vi "Test_LogtoNestedGlobalLogInstance_LogCapturedInGlobalLog.vi"(8 "error in (no error)":errorcluster, 11 "TestCase in":refnum<class "TestComposedLog.lvclass">) -> (0 "error out":errorcluster, 3 "TestCase out":refnum<class "TestComposedLog.lvclass">)   [LabVIEW 2017, in "TestComposedLog.lvclass"]
uses:
  TestComposedLog.lvclass
  Source/Composed Log/Types/Log Level.ctl
  Source/LVQueue Sink/LVQueue Sink.lvclass/LVQueue Sink.ctl
  Source/Composed Log/LoggerReference/LoggerReference.lvclass/LoggerReference.ctl
  26ac907e-b197-4f92-b50b-edca335a3ee8.vi
  26ac907e-b197-4f92-b50b-edca335a3ee8.vi/98f69271-1de1-4081-8ac1-8b840b0807ac.vi
  Source/Composed Log/Singleton Event Log/Get Nested Global Log Instance.vi/b2f05d58-65df-4e80-8f90-78513ac31376.vi
  Source/Composed Log/LoggerReference/Log.vi
  Source/Composed Log/LoggerReference/Get Valid Event Time.vi
  Source/Composed Log/LoggerReference/Return Aggregate Queues.vi
  Source/Composed Log/LoggerReference/Add Aggregate Log.vi
  26ac907e-b197-4f92-b50b-edca335a3ee8.vi/98f69271-1de1-4081-8ac1-8b840b0807ac.vi/bbd2f978-e444-4445-9202-4eeb40a61ae4.vi
  Source/Composed Log/Singleton Event Log/Get Nested Global Log Instance.vi/b2f05d58-65df-4e80-8f90-78513ac31376.vi/e1ecde32-be62-4caa-aa7a-1c02d969ae2d.vi
  Source/Composed Log/LoggerReference/Remove Stale Logs.vi
  Source/Composed Log/LoggerReference/Send Add Sink.vi
  Source/LVQueue Sink/LVQueue Sink.lvclass
  C:/CS/Internal/LabVIEW/Logger/Source/Composed Log/Log Sink/Log Sink.lvclass
  Source/Composed Log/Application Logger/Launch Worker Loop.vi
  Source/Composed Log/LoggerReference/Initialize Logger Instance.vi
  Source/Composed Log/Singleton Event Log/Logger Queue FGV.vi
  Source/Composed Log/Singleton Event Log/Shared Instance FGV.vi
  Source/Composed Log/IErrorFormat/IErrorFormat.lvclass
  Source/Composed Log/LoggerReference/LoggerReference.lvclass
  Source/Composed Log/Log Sink/Log Sink.lvclass
  <vilib>/addons/_JKI Toolkits/VI Tester/TestCase.llb/TestCase.lvclass
  Source/Composed Log/Composed Log.lvlib
  Source/Composed Log/Singleton Event Log/Singleton Event Log.lvlib
  C:/Program Files (x86)/National Instruments/LabVIEW 2017/vi.lib/addons/_JKI Toolkits/VI Tester/TestCase.llb/TestCase.lvclass
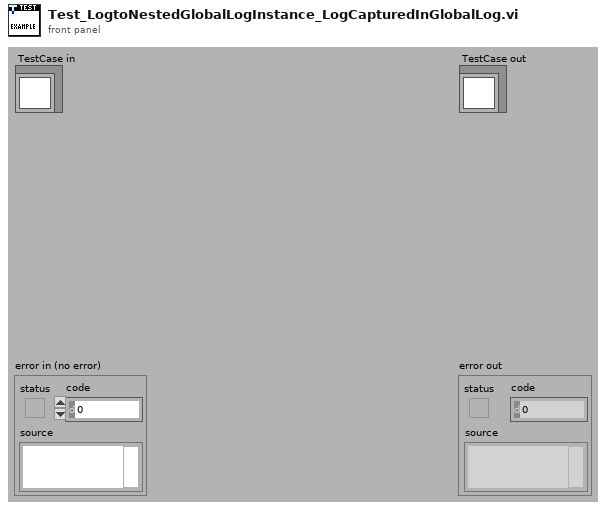
[diagram p1: front panel]
types:
  T1 = typedef "Composed Log.lvlib/Log Level.ctl" = enum16{"Debug", "Info", "Warning", "Error", "Critical"}
  T2 = typedef "Composed Log.lvlib/Log Packet.ctl" = cluster{"Data To Log":string, "Source":string, "Event Level":T1, "Event Time":timestamp}
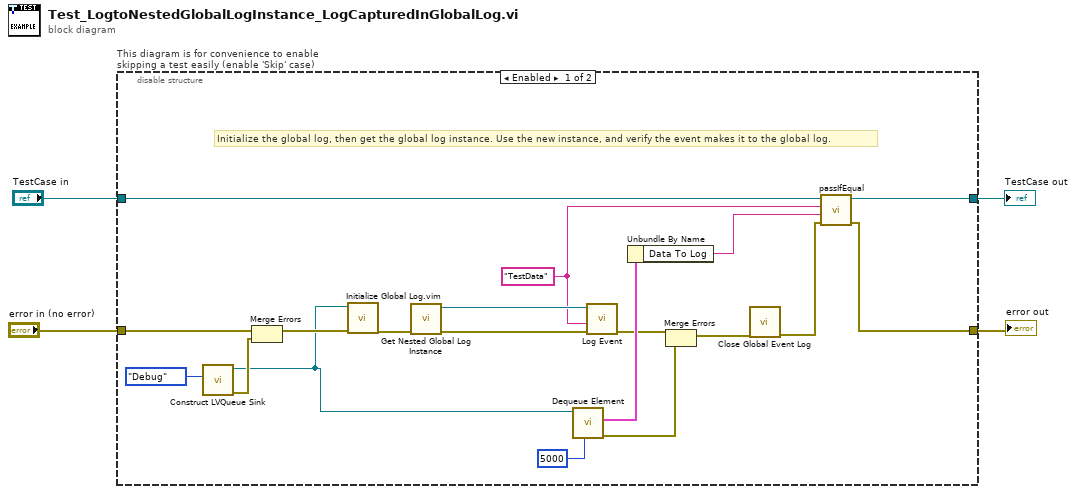
[diagram p0: block diagram]
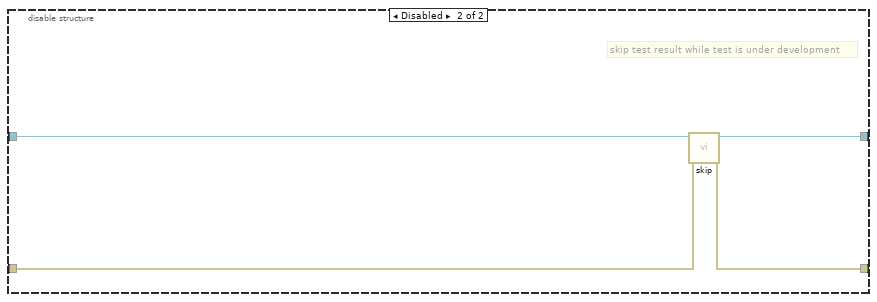
[diagram p2: hidden frame]
diagram:
  n1 = disable-structure "This diagram is for convenience to enable skipping a test easily (enable 'Skip' case)" shown="Enabled" {
    disable-tunnel: "TestCase in" -> [w18 w27]
    disable-tunnel: [w15 w25] -> w1
    disable-tunnel: [w16 w26] -> w3
    disable-tunnel: "error in (no error)" -> [w23 w24]
    frame Enabled {
      w6 = "TestData" ("Data To Log")
      # "Initialize the global log, then get the global log instance. Use the new instance, and verify the event makes it to the global log."
      n2 = call "Construct LVQueue Sink.vi"("LogLevel"=Log_Level."Debug") -> ("error out"=w21:errorcluster, "LVQueue Sink out"=w13:refnum<class "LVQueue Sink.lvclass">)  [unwired: 9 in]
      n3 = Merge Errors(w23, w21) -> (w20:errorcluster)
      n4 = call "Initialize Global Log.vim"("error in (no error)"=w20, "Log Sink(s)"=w13) -> ("error out"=w19:errorcluster)  [unwired: 8 in, 1 out]
      n5 = call "Get Nested Global Log Instance.vi"("error in (no error)"=w19) -> ("error out"=w8:errorcluster, "Nested Global Log Instance Reference"=w7:refnum<class "LoggerReference.lvclass">)  [unwired: 9 in]
      n6 = call "Dequeue Element.vi"("timeout in ms (-1)"=5000, "LVQueue Sink in"=w13) -> ("error out"=w9:errorcluster, "Log Packet"=w12:T2)  [unwired: 6 in, 2 out]
      n7 = call "Log Event.vi"("error in (no error)"=w8, "Data To Log"=w6, "Log Instance"=w7) -> ("error out"=w5:errorcluster)  [unwired: 7 in, 1 out]
      n8 = Unbundle By Name(w12) -> ("Data To Log"=w11:string)
      n9 = Merge Errors(w5, w9) -> (w10:errorcluster)
      n10 = call "Close Global Event Log.vi"("error in (no error)"=w10) -> ("error out"=w17:errorcluster)  [unwired: 10 in]
      n11 = call-dynamic "passIfEqual.vi"("error in (no error)"=w17, "y"=w11, "x"=w6, "TestCase in"=w18) -> ("error out"=w16:errorcluster, "TestCase out"=w15:refnum<class "TestComposedLog.lvclass">)  [unwired: 6 in]
    }
    frame Disabled {
      # "skip test result while test is under development"
      n12 = call <vilib>:"skip.vi"("error in (no error)"=w24, "TestCase in"=w27) -> ("error out"=w26:errorcluster, "TestCase out"=w25:refnum<class "TestComposedLog.lvclass">)  [unwired: 8 in]
    }
  }
  "error out" <- w3
  "TestCase out" <- w1
